vi "Switch Present (Set).vi"(6 "ISOBUS address":T3=-1 caption="ISOBUS address (-1)", 8 "error in":errorcluster, 10 "Switch Present":string, 11 "Mercury Reference In":T4) -> (0 "error out":errorcluster, 2 "Response":T1, 3 "Mercury Reference Out":T4, 4 "Valid?":T2)   [LabVIEW 2019, in "Mercury iXX.lvlib" / "Magnet.lvlib"]
doc: "Set if the switch is present.\n\nNB: The instrument must be in Engineering mode to set this item."
uses:
  Magnet.lvlib
  Controls/Mercury Reference.ctl
  CryoTUM_20210311/sub_vi-s/Equipment/Mercury iXX/Public/Controls/Comms Transport Layer.ctl
  Private/Controls/Query Dynamic Reference.ctl
  Controls/ISOBus Address.ctl
  Controls/Is Valid LED.ctl
  Controls/Response String.ctl
  Private/Controls/Command Verbs.ctl
  mercury/Mercury iXX.lvlib
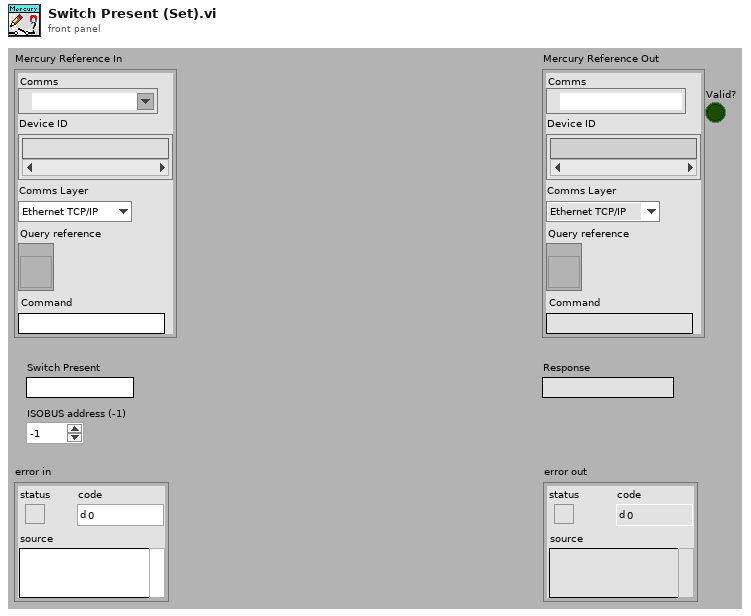
[diagram p1: front panel]
types:
  T1 = typedef "Mercury iXX.lvlib/Response String.ctl" = string
  T2 = typedef "Mercury iXX.lvlib/Is Valid LED.ctl" = bool
  T3 = typedef "Mercury iXX.lvlib/ISOBus Address.ctl" = i32
  T4 = typedef "Mercury iXX.lvlib/Mercury Reference.ctl" = cluster{"Comms":refnum<visa-resource-name>, "Device ID":string[], "Comms Layer":T5, "Command":string, "Query reference":T6}
  T5 = typedef "Mercury iXX.lvlib/Comms Transport Layer.ctl" = enum16{"Ethernet TCP/IP", "USB", "ISOBus - RS-232", "GPIB"}
  T6 = typedef "Mercury iXX.lvlib/Query Dynamic Reference.ctl" = refnum<vi>
  T7 = typedef "Mercury iXX.lvlib/Command Verbs.ctl" = string
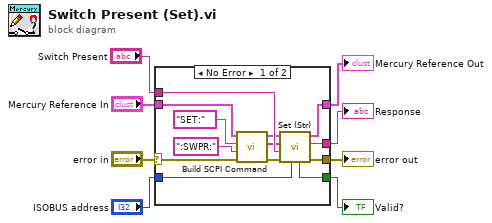
[diagram p0: block diagram]
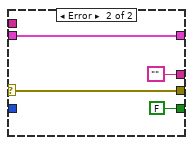
[diagram p2: hidden frame]
diagram:
  n1 = case shown="No Error" "error in" {
    selector: "error in" -> [w15 w24]
    tunnel: "Mercury Reference In" -> [w14 w25]
    tunnel: [w21 w25] -> w7
    tunnel: [w20 w24] -> w6
    tunnel: "ISOBUS address" -> [w19 _]
    tunnel: [w18 T2 FALSE ("Valid?")] -> w4
    tunnel: [w17 ""] -> w3
    tunnel: "Switch Present" -> [w16 _]
    frame No Error {
      n2 = call "Build SCPI Command.vi"("error in"=w15, "Noun(s)"=":SWPR:" ("Command"), "Verb"=T7 "SET:", "Mercury Reference In"=w14) -> ("error out"=w9:errorcluster, "SCPI Message(s)"=w11:string[], "Mercury Reference Out"=w10:T4)  [unwired: 5 out]
      n3 = call "Set (Str).vi"("ISOBUS address"=w19, "error in"=w9, "Command Value (Str)"=w16, "SCPI Message(s)"=w11, "Mercury Reference In"=w10) -> ("error out"=w20:errorcluster, "Response"=w17:T1, "Mercury Reference Out"=w21:T4, "Valid?"=w18:T2)  [unwired: 3 out]
    }
    frame Error {
    }
  }
  "Mercury Reference Out" <- w7
  "error out" <- w6
  "Valid?" <- w4
  "Response" <- w3
